vi "FSK_Spectrum.vi"(8 "error in (no error)":errorcluster caption="错误输入（无错误）", 10 "input_data":cdb[](array[numeric]), 11 "PathIn":path) -> (0 "error out":errorcluster caption="错误输出", 1 "w":dbl[](array[numeric]) format="%#_13g", 2 "output_data":cdb[](array[numeric]) format="%#_13g", 3 "PathOut":path, 4 "SendSig_F":dbl[](array[numeric]) format="%#_13g")   [LabVIEW 2015]
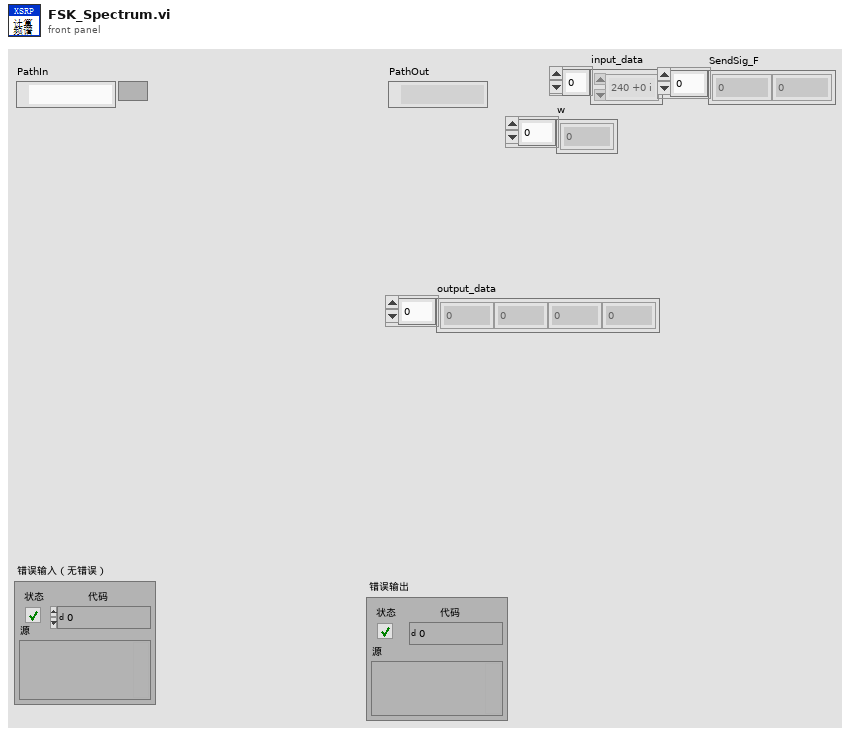
[diagram p1: front panel]
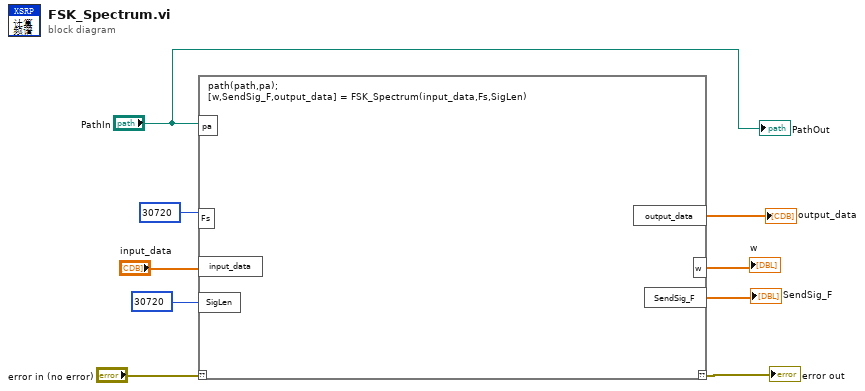
[diagram p0: block diagram]
diagram:
  n1 = script code="path(path,pa);\n[w,SendSig_F,output_data] = FSK_Spectrum(input_data,Fs,SigLen)"("??"="error in (no error)", "pa"="PathIn", "input_data"="input_data", "SigLen"=30720, "Fs"=30720) -> ("??"=→"error out":errorcluster, "output_data"=→"output_data":cdb[], "w"=→"w":dbl[], "SendSig_F"=→"SendSig_F":dbl[])
  "PathOut" <- "PathIn"
